vi "Variable@Arange__Parameter.vi"(1 "ParamterIn":string) -> (0 "ParamterOut":string)   [LabVIEW 2020]
panel:
  in  "Step":string(combo)
  in  "End":string(combo)
  in  "Section":string(combo)
  in  "Start":string(combo)
  in  "ParameterName":string(combo)
  in  "Confirm":bool
  # "Variable@Arange $Variable,$Start,$End,$Step(,$Section)\nEX: test,0,10,1   -> [0;1;2;3;4;5;6;7;8;9]"
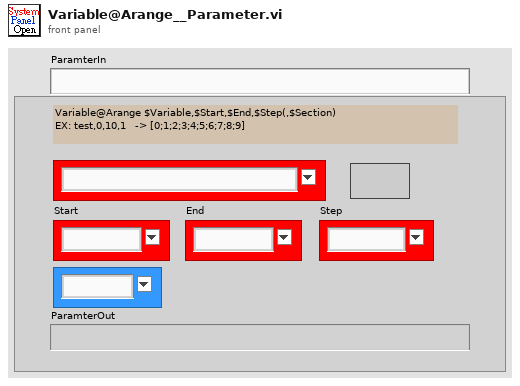
[diagram p1: front panel]
types:
  T1 = enum16{"Get", "Init", "Set", "Delete", "GetElement", "Inc", "Dec", "ReName"}
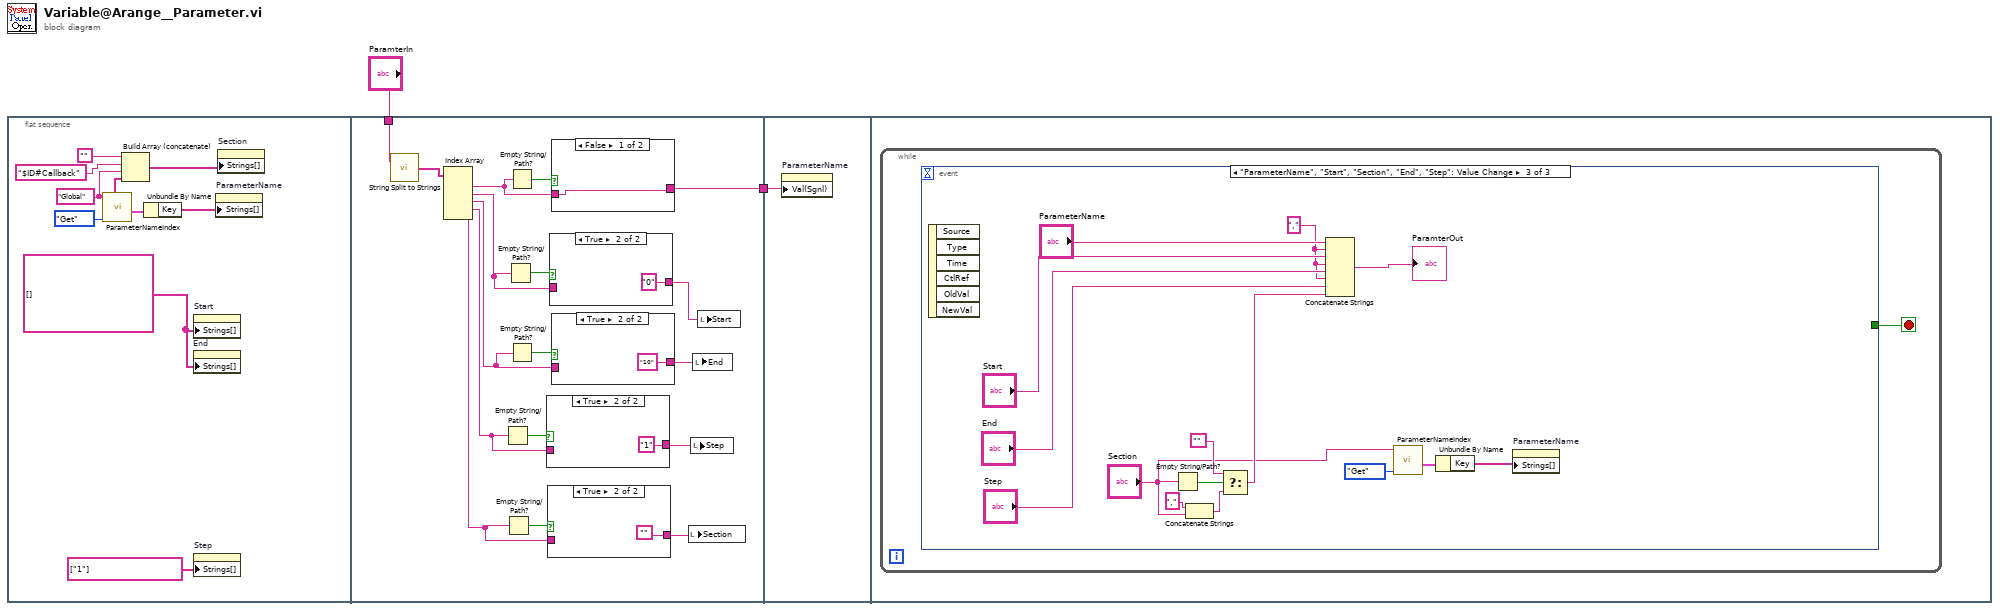
[diagram p0: block diagram]
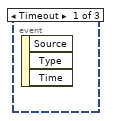
[diagram p7: hidden frame]
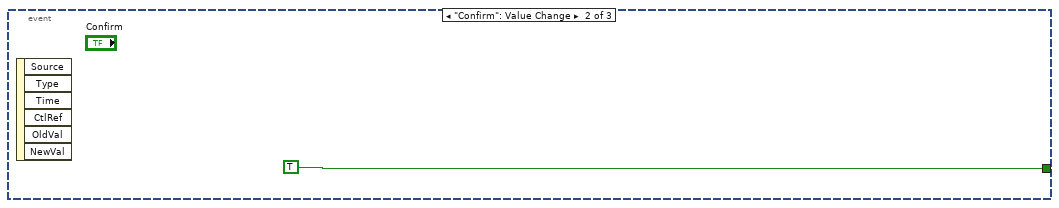
[diagram p8: hidden frame]
diagram:
  n1 = flat-sequence {
    tunnel: "ParamterIn" -> [w25]
    tunnel: [w27] -> w1
    tunnel: w1 -> [w40]
    frame #0 {
      w5 = "Global" ("VariableSection")
      w9 = string[] [] ("Strings []")
      n2 = call "ParameterNameIndex.vi"("OP"=T1."Get", "VariableSection"=w5) -> ("GlobalKeyValue"=w12:cluster{"Key":string[], "Value":string[]}, "SectionList"=w6:string[])  [unwired: 3 in, 5 out]
      n3 = Build Array (concatenate)("", "$ID#Callback" ("VariableSection"), w5, w6) -> (w4:string[])
      n4 = Unbundle By Name(w12) -> ("Key"=w11:string[])
      n5 = property on="Start" class="CmbBox"("Strings[]"=w9) -> ()  [unwired: 2 in, 2 out]
      n6 = property on="End" class="CmbBox"("Strings[]"=w9) -> ()  [unwired: 2 in, 2 out]
      n7 = property on="Step" class="CmbBox"("Strings[]"=string[] ["1"] ("Strings []")) -> ()  [unwired: 2 in, 2 out]
      n8 = property on="ParameterName" class="CmbBox"("Strings[]"=w11) -> ()  [unwired: 2 in, 2 out]
      n9 = property on="Section" class="CmbBox"("Strings[]"=w4) -> ()  [unwired: 2 in, 2 out]
    }
    frame #1 {
      n10 = call "String Split to Strings.vi"("String"=w25) -> ("Array"=w24:string[])  [unwired: 1 in]
      n11 = Index Array(array=w24) -> (element #1=w23:string, element #2=w22:string, element #3=w17:string, element #4=w14:string, element #5=w13:string)  [unwired: 5 in]
      n12 = Empty String/Path?(string/path=w14) -> (empty?=w16:bool)
      n13 = Empty String/Path?(string/path=w13) -> (empty?=w21:bool)
      n14 = Empty String/Path?(string/path=w22) -> (empty?=w28:bool)
      n15 = Empty String/Path?(string/path=w23) -> (empty?=w29:bool)
      n16 = Empty String/Path?(string/path=w17) -> (empty?=w19:bool)
      n17 = case shown="True" w16 {
        tunnel: w14 -> [w30 _]
        tunnel: [w30 "1"] -> w15
        frame False {
        }
        frame True {
        }
      }
      n18 = case shown="True" w21 {
        tunnel: w13 -> [w34 _]
        tunnel: [w34 ""] -> w20
        frame False {
        }
        frame True {
        }
      }
      n19 = case shown="True" w28 {
        tunnel: w22 -> [w36 _]
        tunnel: [w36 "0"] -> w26
        frame False {
        }
        frame True {
        }
      }
      n20 = case shown="False" w29 {
        tunnel: w23 -> [w38 w39]
        tunnel: [w38 w39] -> w27
        frame False {
        }
        frame True {
        }
      }
      n21 = case shown="True" w19 {
        tunnel: w17 -> [w32 _]
        tunnel: [w32 "10"] -> w18
        frame False {
        }
        frame True {
        }
      }
      n22 = local write "Section"(w20) -> ()
      n23 = local write "Step"(w15) -> ()
      n24 = local write "End"(w18) -> ()
      n25 = local write "Start"(w26) -> ()
    }
    frame #2 {
      n26 = property on="ParameterName" class="CmbBox"("Val(Sgnl)"=w40) -> ()  [unwired: 2 in, 2 out]
    }
    frame #3 {
      n27 = while {
        stop <- w41 stop-if-true
        n28 = event shown="[2] \"ParameterName\", \"Start\", \"Section\", \"End\", \"Step\": Value Change" {
          selector: _ -> [_ _ _]
          dyn-events: _ -> [_ _ _]
          timeout: _ -> [_ _ _]
          tunnel: [_ TRUE _] -> w41
          event Timeout {
            n29 = event-data() -> ()  [unwired: 1 in, 3 out]
          }
          event "Confirm": Value Change {
            n30 = event-data() -> ()  [unwired: 1 in, 6 out]
          }
          event "ParameterName", "Start", "Section", "End", "Step": Value Change {
            w48 = "," ("string")
            n31 = event-data() -> ()  [unwired: 1 in, 6 out]
            n32 = Empty String/Path?(string/path="Section") -> (empty?=w53:bool)
            n33 = Concatenate Strings("," ("string"), "Section") -> (w54:string)
            n34 = Select(t="", s=w53, f=w54) -> (s? t:f=w46:string)
            n35 = Concatenate Strings("ParameterName", w48, "Start", w48, "End", w48, "Step", w46) -> (→"ParamterOut":string)
            n36 = call "ParameterNameIndex.vi"("OP"=T1."Get", "VariableSection"="Section") -> ("GlobalKeyValue"=w44:cluster{"Key":string[], "Value":string[]})  [unwired: 3 in, 6 out]
            n37 = Unbundle By Name(w44) -> ("Key"=w52:string[])
            n38 = property on="ParameterName" class="CmbBox"("Strings[]"=w52) -> ()  [unwired: 2 in, 2 out]
          }
        }
      }
    }
  }
